vi "test-Diff-Drive-Accel-Limiter-Test1.vi"(8 "error in (no error)":errorcluster) -> (0 "error out":errorcluster, 3 "All tests passed":bool)   [LabVIEW 2019]
uses:
  <vilib>/Rock Robotics/WPI/ThirdParty/JAS_Junk/TrajLib/Trajectory_Library.lvlib
  <vilib>/Analysis/NI_AALBase.lvlib
  <vilib>/Analysis/baseanly.llb/Real A x B.vi
  <vilib>/Analysis/Matrix/NI_Matrix.lvlib
  <vilib>/Analysis/Matrix/Numeric/Add/Add - RM,RM.vi
panel:
  out "max value 6":dbl
  out "max value 5":dbl
  out "max value 4":dbl
  out "max value 3":dbl
  out "max value 2":dbl
  out "max value":dbl
  out "Test 1":bool
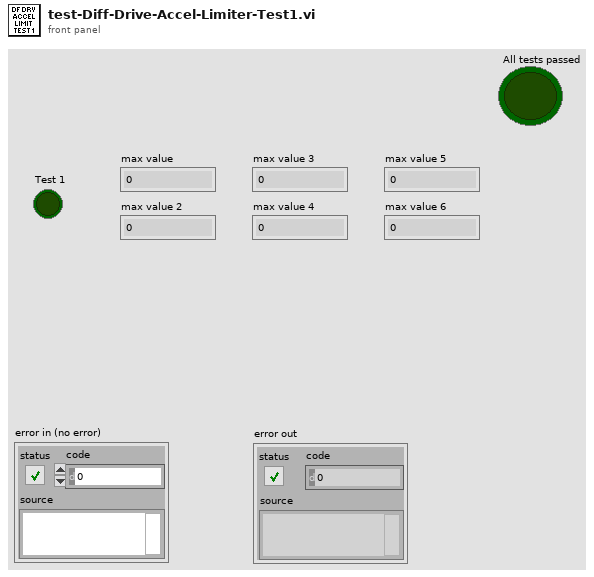
[diagram p1: front panel]
types:
  T1 = typedef "NI_Matrix.lvlib/RealMatrix.ctl" = dbl[][]
  T2 = typedef "Trajectory_Library.lvlib/LINEAR_SYSTEM.ctl" = cluster{"m_A":T1, "m_B":T1, "m_C":T1, "m_D":T1, "States":i32, "Inputs":i32, "Outputs":i32}
  T3 = typedef "Trajectory_Library.lvlib/DIFF_DRIVE_ACCEL_LIMIT.ctl" = cluster{"m_system":T2, "m_trackwidth":dbl, "m_maxLinearAccel":dbl, "m_maxAngularAccel":dbl, "m_minLinearAccel":dbl}
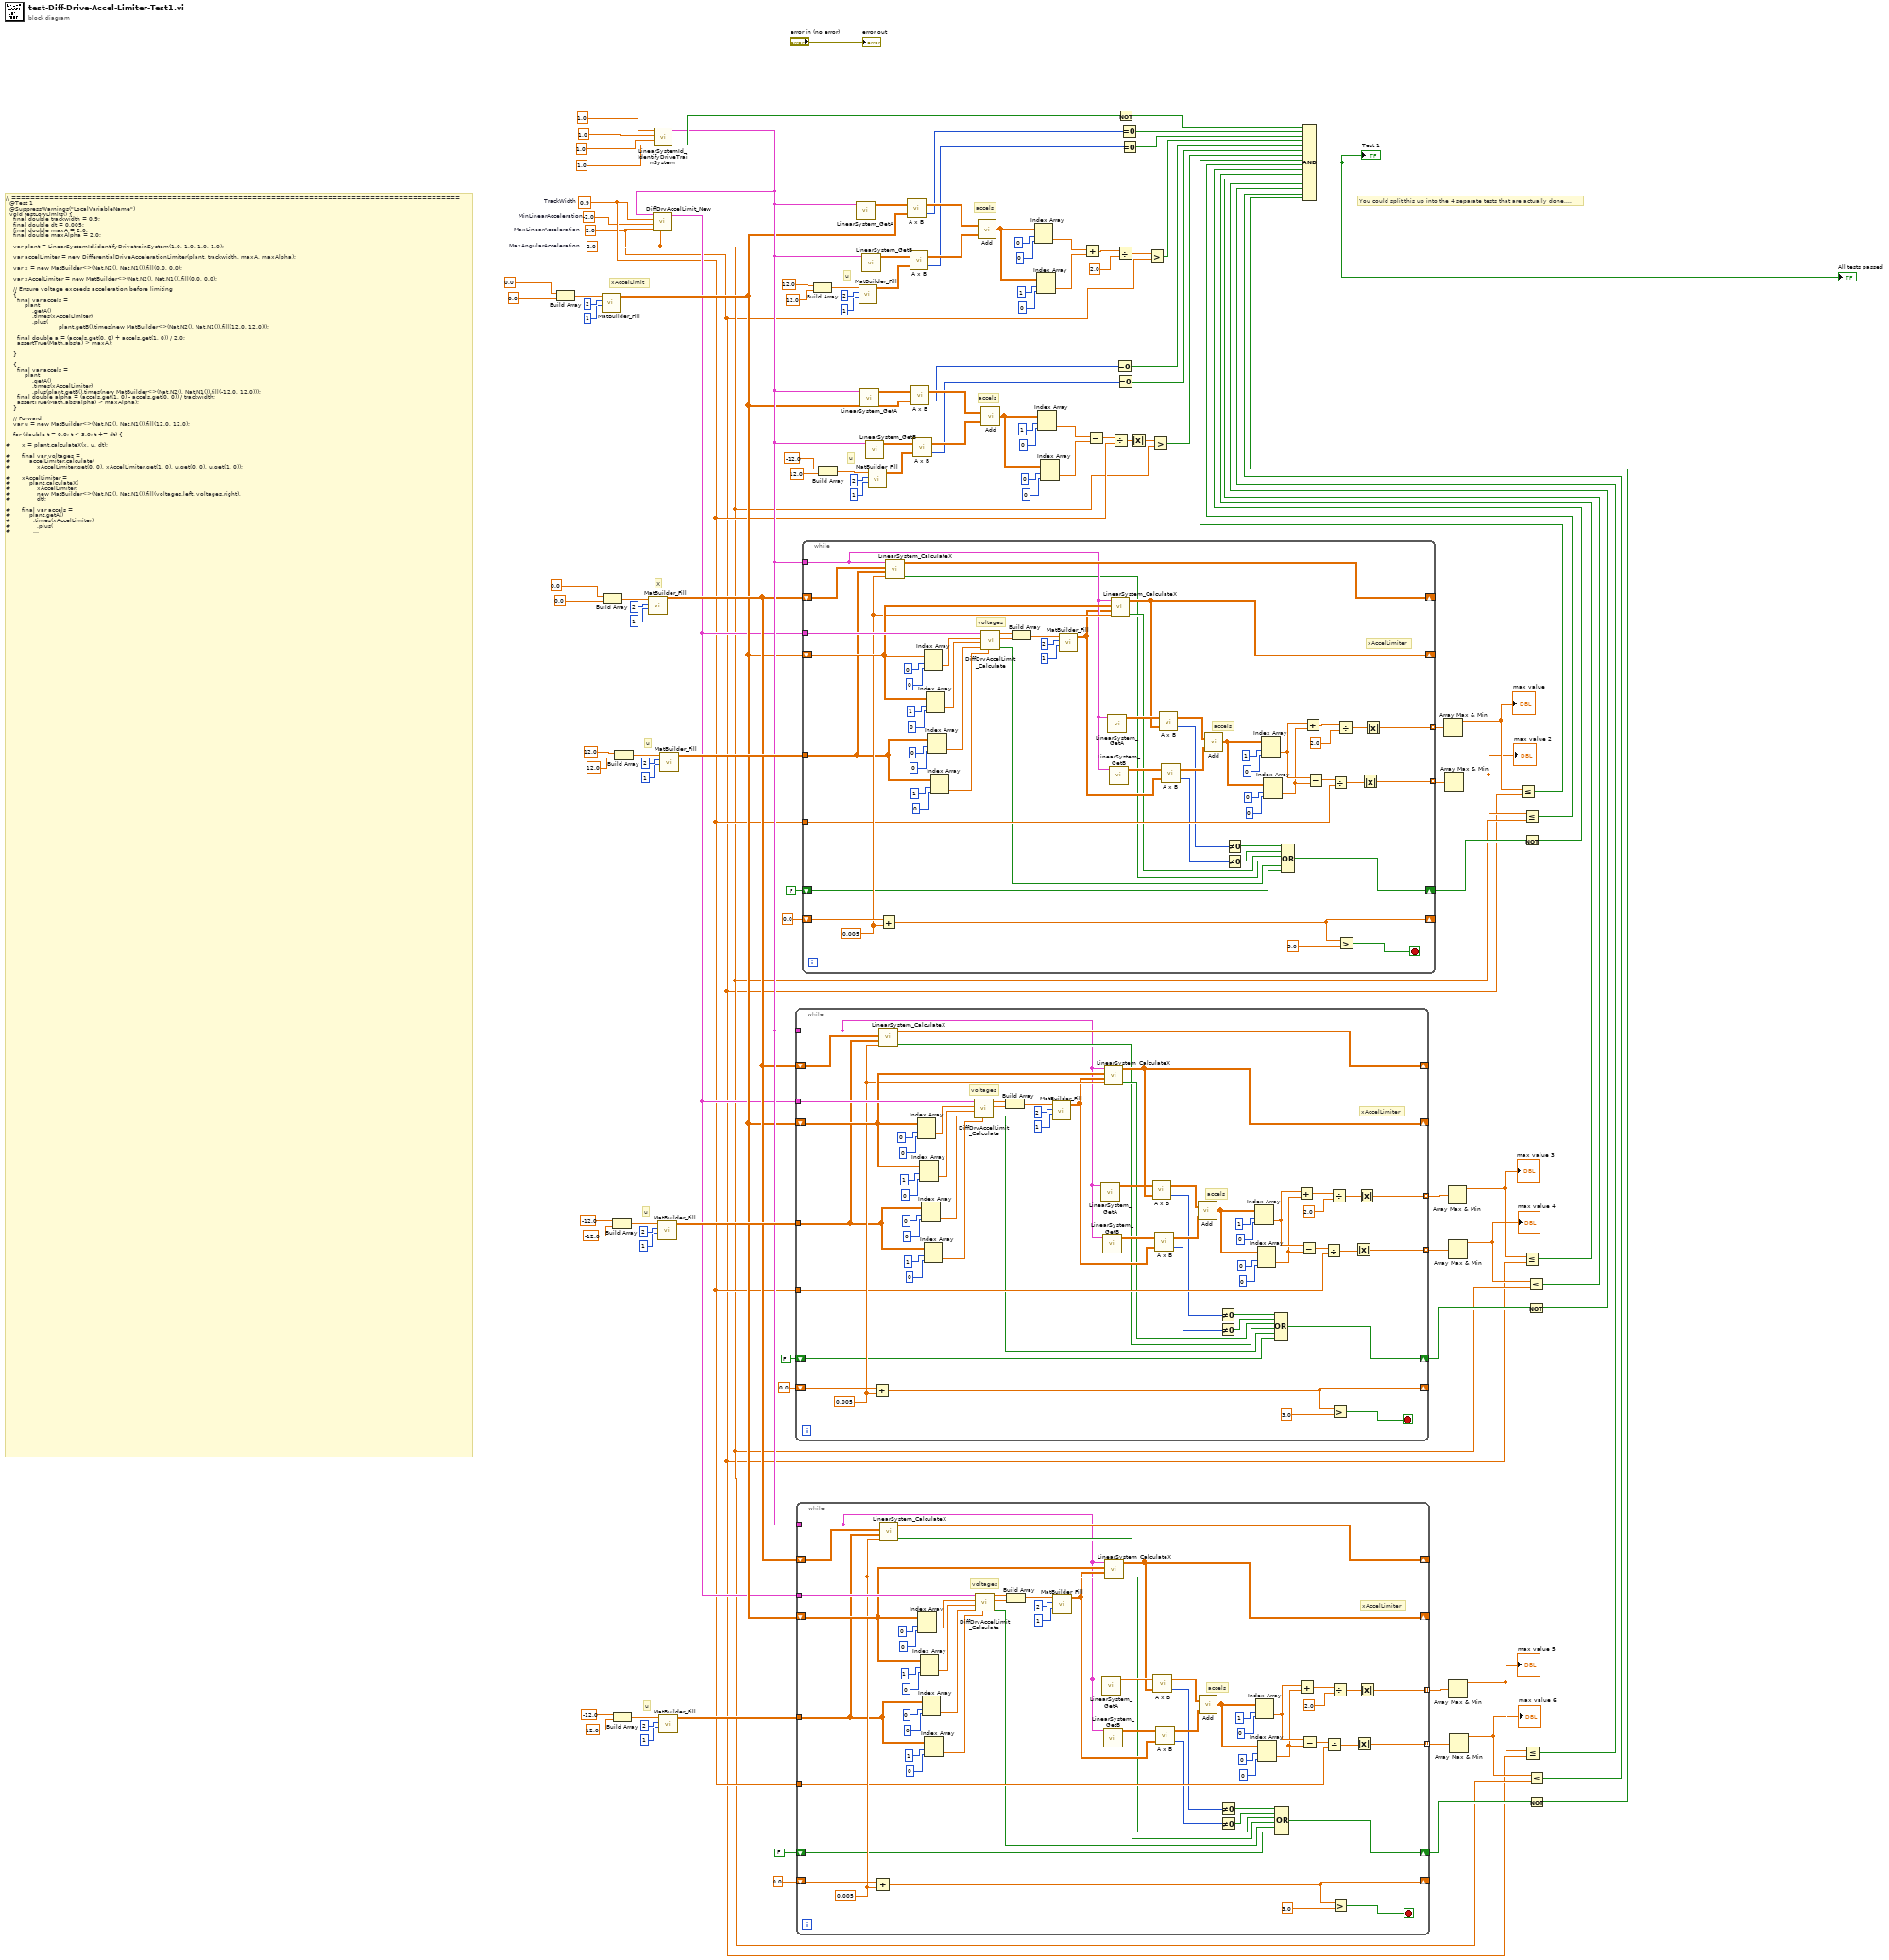
[diagram p0: block diagram]
diagram:
  w1 = -2.0  # MinLinearAcceleration
  w8 = 0.9  # TrackWidth
  w2 = 2.0  # MaxLinearAcceleration
  w3 = 2.0  # MaxAngularAcceleration
  # "You could split this up into the 4 separate tests that are actually done...."
  # "u"
  # "u"
  # "u"
  # "u"
  # "u"
  # "accels"
  # "accels"
  # "xAccelLimit"
  # "X"
  # "// ===============================================================================================\n  @Test 1\n  @SuppressWarnings(\"LocalVariableName\")\n  void testLowLimits() {\n    final double trackwidth = 0.9;\n    final double dt = 0.005;\n    final double maxA = 2.0;\n    final double maxAlpha = 2.0;\n\n    var plant = LinearSystemId.identifyDrivetrainSystem(1.0, 1.0, 1.0, 1.0);\n\n    var accelLimiter = new DifferentialDriveAccelerationLimiter(plant, trackwidth, maxA, maxAlpha);\n\n    var x = new MatBuilder<>(Nat.N2(), Nat.N1()).fill(0.0, 0.0);\n\n    var xAccelLimiter = new MatBuilder<>(Nat.N2(), Nat.N1()).fill(0.0, 0.0);\n\n    // Ensure voltage exceeds acceleration before limiting\n    {\n      final var accels =\n          plant\n              .getA()\n              .times(xAccelLimiter)\n              .plus(\n                            plant.getB().times(new MatBuilder<>(Nat.N2(), Nat.N1()).fill(12.0, 12.0)));\n\n      final double a = (accels.get(0, 0) + accels.get(1, 0)) / 2.0;\n      assertTrue(Math.abs(a) > maxA);\n\n    }\n\n    {\n      final var accels =\n          plant\n              .getA()\n              .times(xAccelLimiter)\n              .plus(plant.getB().times(new MatBuilder<>(Nat.N2(), Nat.N1()).fill(-12.0, 12.0)));\n      final double alpha = (accels.get(1, 0) - accels.get(0, 0)) / trackwidth;\n      assertTrue(Math.abs(alpha) > maxAlpha);\n    }\n\n    // Forward\n    var u = new MatBuilder<>(Nat.N2(), Nat.N1()).fill(12.0, 12.0);\n\n    for (double t = 0.0; t < 3.0; t += dt) {\n\n#      x = plant.calculateX(x, u, dt);\n\n#      final var voltages =\n#          accelLimiter.calculate(\n#              xAccelLimiter.get(0, 0), xAccelLimiter.get(1, 0), u.get(0, 0), u.get(1, 0));\n\n#      xAccelLimiter =\n#          plant.calculateX(\n#              xAccelLimiter,\n#              new MatBuilder<>(Nat.N2(), Nat.N1()).fill(voltages.left, voltages.right),\n#              dt);\n\n#      final var accels =\n#          plant.getA()\n#            .times(xAccelLimiter)\n#              .plus(\n#                  plant.getB()\n#                      .times(\n#                          new MatBuilder<>(Nat.N2(), Nat.N1())\n#                              .fill(voltages.left, voltages.right)));\n\n#      final double a = (accels.get(0, 0) + accels.get(1, 0)) / 2.0;\n\n#      final double alpha = (accels.get(1, 0) - accels.get(0, 0)) / trackwidth;\n\n#      assertTrue(Math.abs(a) <= maxA);\n#      assertTrue(Math.abs(alpha) <= maxAlpha);\n\n#    }\n\n    // Backward\n    u = new MatBuilder<>(Nat.N2(), Nat.N1()).fill(-12.0, -12.0);\n\n    for (double t = 0.0; t < 3.0; t += dt) {\n      x = plant.calculateX(x, u, dt);\n      final var voltages =\n          accelLimiter.calculate(\n              xAccelLimiter.get(0, 0), xAccelLimiter.get(1, 0), u.get(0, 0), u.get(1, 0));\n      xAccelLimiter =\n          plant.calculateX(\n              xAccelLimiter,\n              new MatBuilder<>(Nat.N2(), Nat.N1()).fill(voltages.left, voltages.right),\n              dt);\n\n      final var accels =\n          plant\n              .getA()\n              .times(xAccelLimiter)\n              .plus(\n                  plant\n                      .getB()\n                      .times(\n                          new MatBuilder<>(Nat.N2(), Nat.N1())\n                              .fill(voltages.left, voltages.right)));\n\n      final double a = (accels.get(0, 0) + accels.get(1, 0)) / 2.0;\n\n      final double alpha = (accels.get(1, 0) - accels.get(0, 0)) / trackwidth;\n\n      assertTrue(Math.abs(a) <= maxA);\n      assertTrue(Math.abs(alpha) <= maxAlpha);\n    }\n\n\n    // Rotate CCW\n    u = new MatBuilder<>(Nat.N2(), Nat.N1()).fill(-12.0, 12.0);\n    for (double t = 0.0; t < 3.0; t += dt) {\n      x = plant.calculateX(x, u, dt);\n      final var voltages =\n          accelLimiter.calculate(\n              xAccelLimiter.get(0, 0), xAccelLimiter.get(1, 0), u.get(0, 0), u.get(1, 0));\n      xAccelLimiter =\n          plant.calculateX(\n              xAccelLimiter,\n              new MatBuilder<>(Nat.N2(), Nat.N1()).fill(voltages.left, voltages.right),\n              dt);\n\n      final var accels =\n          plant\n              .getA()\n              .times(xAccelLimiter)\n              .plus(\n                  plant\n                      .getB()\n                      .times(\n                          new MatBuilder<>(Nat.N2(), Nat.N1())\n                              .fill(voltages.left, voltages.right)));\n      final double a = (accels.get(0, 0) + accels.get(1, 0)) / 2.0;\n      final double alpha = (accels.get(1, 0) - accels.get(0, 0)) / trackwidth;\n      assertTrue(Math.abs(a) <= maxA);\n      assertTrue(Math.abs(alpha) <= maxAlpha);\n    }\n  }"
  n1 = Build Array(0.0 ("element"), 0.0 ("element")) -> (w114:dbl[])
  n2 = call <vilib>:"MatBuilder_Fill.vi"("Columns"=1, "Rows"=2, "Value List"=w114) -> ("output matrix"=w10:T1)  [unwired: 8 in]
  n3 = Build Array(0.0 ("element"), 0.0 ("element")) -> (w119:dbl[])
  n4 = Build Array(-12.0 ("element"), -12.0 ("element")) -> (w39:dbl[])
  n5 = Build Array(-12.0 ("element"), 12.0 ("element")) -> (w23:dbl[])
  n6 = Build Array(12.0 ("element"), 12.0 ("element")) -> (w57:dbl[])
  n7 = call <vilib>:"MatBuilder_Fill.vi"("Columns"=1, "Rows"=2, "Value List"=w119) -> ("output matrix"=w11:T1)  [unwired: 8 in]
  n8 = call <vilib>:"LinearSystemId_IdentifyDriveTrainSystem.vi"("kAAngular"=1.0 ("rbMeters"), "kVAngular"=1.0 ("rMeters"), "kALinear"=1.0 ("MassKg"), "kVLinear"=1.0 ("JKgMetersSquared")) -> ("Size Coerced"=w94:bool, "Linearsystem"=w12:T2)  [unwired: 6 in]
  n9 = call <vilib>:"DiffDrvAccelLimit_New.vi"("MaxAngularAcceleration"=w3, "MaxLinearAcceleration"=w2, "MinLinearAcceleration"=w1, "TrackWidth"=w8, "LINEARSYSTEM"=w12) -> ("outDiffDriveAccelLimit"=w9:T3)  [unwired: 5 in, 1 out]
  n10 = call <vilib>:"MatBuilder_Fill.vi"("Columns"=1, "Rows"=2, "Value List"=w39) -> ("output matrix"=w34:T1)  [unwired: 8 in]
  n11 = call <vilib>:"MatBuilder_Fill.vi"("Columns"=1, "Rows"=2, "Value List"=w23) -> ("output matrix"=w18:T1)  [unwired: 8 in]
  n12 = call <vilib>:"MatBuilder_Fill.vi"("Columns"=1, "Rows"=2, "Value List"=w57) -> ("output matrix"=w51:T1)  [unwired: 8 in]
  n13 = while {
    shift-right: [w179] -> _
    shift-left: 0.0 -> [w182]
    tunnel: w34 -> [w140]
    shift-right: [w172] -> _
    shift-left: w11 -> [w178]
    tunnel: w9 -> [w177]
    shift-right: [w147] -> _
    shift-left: w10 -> [w163]
    tunnel: w8 -> [w139]
    tunnel: [w136] -> w31 mode=indexing
    tunnel: [w135] -> w30 mode=indexing
    shift-right: [w126] -> w29
    shift-left: FALSE -> [w127]
    tunnel: w12 -> [w125]
    stop <- w181 stop-if-true
    w157 = 0.005
    # "voltages"
    # "xAccelLimiter"
    # "accels"
    n14 = Add(x=w182, y=w157) -> (x+y=w179:dbl)
    n15 = call <vilib>:"LinearSystem_CalculateX.vi"("dT_Seconds"=w157, "ClampedU"=w140, "X"=w178, "Linearsystem"=w125) -> ("Error"=w129:bool, "outX"=w172:T1)  [unwired: 6 in]
    n16 = Index Array(array=w163, index (row)=0, index (col)=0) -> (element=w171:dbl)
    n17 = Index Array(array=w163, index (row)=1, index (col)=0) -> (element=w170:dbl)
    n18 = Index Array(array=w140, index (row)=0, index (col)=0) -> (element=w165:dbl)
    n19 = Index Array(array=w140, index (row)=1, index (col)=0) -> (element=w164:dbl)
    n20 = call <vilib>:"DiffDrvAccelLimit_Calculate.vi"("RightVoltage"=w164, "LeftVoltage"=w165, "RightVelocity"=w170, "LeftVelocity"=w171, "inDiffDriveAccelLimit"=w177) -> ("Error"=w128:bool, "NewRightVoltage"=w158:dbl, "NewLeftVoltage"=w159:dbl)  [unwired: 4 in]
    n21 = Build Array(w159, w158) -> (w162:dbl[])
    n22 = call <vilib>:"MatBuilder_Fill.vi"("Columns"=1, "Rows"=2, "Value List"=w162) -> ("output matrix"=w146:T1)  [unwired: 8 in]
    n23 = call <vilib>:"LinearSystem_GetA.vi"("Linearsystem"=w125) -> ("A"=w156:T1)  [unwired: 10 in]
    n24 = call <vilib>:"LinearSystem_GetB.vi"("Linearsystem"=w125) -> ("B"=w155:T1)  [unwired: 10 in]
    n25 = call <vilib>:"LinearSystem_CalculateX.vi"("dT_Seconds"=w157, "ClampedU"=w146, "X"=w163, "Linearsystem"=w125) -> ("Error"=w130:bool, "outX"=w147:T1)  [unwired: 6 in]
    n26 = call-poly <vilib>:"A x B.vi"("B"=w147, "A"=w156) -> ("error"=w133:i32, "A x B"=w154:T1)
    n27 = call-poly <vilib>:"A x B.vi"("B"=w146, "A"=w155) -> ("error"=w132:i32, "A x B"=w153:T1)
    n28 = call-poly <vilib>:"Add.vi"("Real Matrix B"=w153, "Real Matrix A"=w154) -> ("A + B"=w148:T1)
    n29 = Not Equal To 0?(x=w133) -> (x != 0?=w134:bool)
    n30 = Not Equal To 0?(x=w132) -> (x != 0?=w131:bool)
    n31 = Index Array(array=w148, index (row)=1, index (col)=0) -> (element=w142:dbl)
    n32 = Index Array(array=w148, index (row)=0, index (col)=0) -> (element=w141:dbl)
    n33 = Compound Arithmetic op=OR(w134, w131, w130, w129, w128, w127) -> (w126:bool)
    n34 = Add(x=w142, y=w141) -> (x+y=w145:dbl)
    n35 = Subtract(x=w142, y=w141) -> (x-y=w143:dbl)
    n36 = Divide(x=w143, y=w139) -> (x/y=w137:dbl)
    n37 = Divide(x=w145, y=2.0) -> (x/y=w138:dbl)
    n38 = Greater?(x=w179, y=3.0) -> (0:w181:bool)
    n39 = Absolute Value(x=w137) -> (abs(x)=w135:dbl)
    n40 = Absolute Value(x=w138) -> (abs(x)=w136:dbl)
  }
  n41 = while {
    shift-right: [w237] -> _
    shift-left: 0.0 -> [w240]
    tunnel: w18 -> [w198]
    shift-right: [w230] -> _
    shift-left: w11 -> [w236]
    tunnel: w9 -> [w235]
    shift-right: [w205] -> _
    shift-left: w10 -> [w221]
    tunnel: w8 -> [w197]
    tunnel: [w194] -> w15 mode=indexing
    tunnel: [w193] -> w14 mode=indexing
    shift-right: [w184] -> w13
    shift-left: FALSE -> [w185]
    tunnel: w12 -> [w183]
    stop <- w239 stop-if-true
    w215 = 0.005
    # "voltages"
    # "xAccelLimiter"
    # "accels"
    n42 = Add(x=w240, y=w215) -> (x+y=w237:dbl)
    n43 = call <vilib>:"LinearSystem_CalculateX.vi"("dT_Seconds"=w215, "ClampedU"=w198, "X"=w236, "Linearsystem"=w183) -> ("Error"=w187:bool, "outX"=w230:T1)  [unwired: 6 in]
    n44 = Index Array(array=w221, index (row)=0, index (col)=0) -> (element=w229:dbl)
    n45 = Index Array(array=w221, index (row)=1, index (col)=0) -> (element=w228:dbl)
    n46 = Index Array(array=w198, index (row)=0, index (col)=0) -> (element=w223:dbl)
    n47 = Index Array(array=w198, index (row)=1, index (col)=0) -> (element=w222:dbl)
    n48 = call <vilib>:"DiffDrvAccelLimit_Calculate.vi"("RightVoltage"=w222, "LeftVoltage"=w223, "RightVelocity"=w228, "LeftVelocity"=w229, "inDiffDriveAccelLimit"=w235) -> ("Error"=w186:bool, "NewRightVoltage"=w216:dbl, "NewLeftVoltage"=w217:dbl)  [unwired: 4 in]
    n49 = Build Array(w217, w216) -> (w220:dbl[])
    n50 = call <vilib>:"MatBuilder_Fill.vi"("Columns"=1, "Rows"=2, "Value List"=w220) -> ("output matrix"=w204:T1)  [unwired: 8 in]
    n51 = call <vilib>:"LinearSystem_GetA.vi"("Linearsystem"=w183) -> ("A"=w214:T1)  [unwired: 10 in]
    n52 = call <vilib>:"LinearSystem_GetB.vi"("Linearsystem"=w183) -> ("B"=w213:T1)  [unwired: 10 in]
    n53 = call <vilib>:"LinearSystem_CalculateX.vi"("dT_Seconds"=w215, "ClampedU"=w204, "X"=w221, "Linearsystem"=w183) -> ("Error"=w188:bool, "outX"=w205:T1)  [unwired: 6 in]
    n54 = call-poly <vilib>:"A x B.vi"("B"=w205, "A"=w214) -> ("error"=w191:i32, "A x B"=w212:T1)
    n55 = call-poly <vilib>:"A x B.vi"("B"=w204, "A"=w213) -> ("error"=w190:i32, "A x B"=w211:T1)
    n56 = call-poly <vilib>:"Add.vi"("Real Matrix B"=w211, "Real Matrix A"=w212) -> ("A + B"=w206:T1)
    n57 = Not Equal To 0?(x=w191) -> (x != 0?=w192:bool)
    n58 = Not Equal To 0?(x=w190) -> (x != 0?=w189:bool)
    n59 = Index Array(array=w206, index (row)=1, index (col)=0) -> (element=w200:dbl)
    n60 = Index Array(array=w206, index (row)=0, index (col)=0) -> (element=w199:dbl)
    n61 = Compound Arithmetic op=OR(w192, w189, w188, w187, w186, w185) -> (w184:bool)
    n62 = Add(x=w200, y=w199) -> (x+y=w203:dbl)
    n63 = Subtract(x=w200, y=w199) -> (x-y=w201:dbl)
    n64 = Divide(x=w201, y=w197) -> (x/y=w195:dbl)
    n65 = Divide(x=w203, y=2.0) -> (x/y=w196:dbl)
    n66 = Greater?(x=w237, y=3.0) -> (0:w239:bool)
    n67 = Absolute Value(x=w195) -> (abs(x)=w193:dbl)
    n68 = Absolute Value(x=w196) -> (abs(x)=w194:dbl)
  }
  n69 = while {
    shift-right: [w295] -> _
    shift-left: 0.0 -> [w298]
    tunnel: w12 -> [w263]
    tunnel: w51 -> [w255]
    shift-right: [w288] -> _
    shift-left: w11 -> [w294]
    tunnel: w9 -> [w293]
    shift-right: [w262] -> _
    shift-left: w10 -> [w279]
    tunnel: w8 -> [w254]
    tunnel: [w251] -> w50 mode=indexing
    tunnel: [w250] -> w49 mode=indexing
    shift-right: [w241] -> w45
    shift-left: FALSE -> [w242]
    stop <- w297 stop-if-true
    w273 = 0.005
    # "voltages"
    # "xAccelLimiter"
    # "accels"
    n70 = Add(x=w298, y=w273) -> (x+y=w295:dbl)
    n71 = call <vilib>:"LinearSystem_CalculateX.vi"("dT_Seconds"=w273, "ClampedU"=w255, "X"=w294, "Linearsystem"=w263) -> ("Error"=w244:bool, "outX"=w288:T1)  [unwired: 6 in]
    n72 = Index Array(array=w279, index (row)=0, index (col)=0) -> (element=w287:dbl)
    n73 = Index Array(array=w279, index (row)=1, index (col)=0) -> (element=w286:dbl)
    n74 = Index Array(array=w255, index (row)=0, index (col)=0) -> (element=w281:dbl)
    n75 = Index Array(array=w255, index (row)=1, index (col)=0) -> (element=w280:dbl)
    n76 = call <vilib>:"DiffDrvAccelLimit_Calculate.vi"("RightVoltage"=w280, "LeftVoltage"=w281, "RightVelocity"=w286, "LeftVelocity"=w287, "inDiffDriveAccelLimit"=w293) -> ("Error"=w243:bool, "NewRightVoltage"=w274:dbl, "NewLeftVoltage"=w275:dbl)  [unwired: 4 in]
    n77 = Build Array(w275, w274) -> (w278:dbl[])
    n78 = call <vilib>:"MatBuilder_Fill.vi"("Columns"=1, "Rows"=2, "Value List"=w278) -> ("output matrix"=w261:T1)  [unwired: 8 in]
    n79 = call <vilib>:"LinearSystem_GetA.vi"("Linearsystem"=w263) -> ("A"=w272:T1)  [unwired: 10 in]
    n80 = call <vilib>:"LinearSystem_GetB.vi"("Linearsystem"=w263) -> ("B"=w271:T1)  [unwired: 10 in]
    n81 = call <vilib>:"LinearSystem_CalculateX.vi"("dT_Seconds"=w273, "ClampedU"=w261, "X"=w279, "Linearsystem"=w263) -> ("Error"=w245:bool, "outX"=w262:T1)  [unwired: 6 in]
    n82 = call-poly <vilib>:"A x B.vi"("B"=w262, "A"=w272) -> ("error"=w248:i32, "A x B"=w270:T1)
    n83 = call-poly <vilib>:"A x B.vi"("B"=w261, "A"=w271) -> ("error"=w247:i32, "A x B"=w269:T1)
    n84 = call-poly <vilib>:"Add.vi"("Real Matrix B"=w269, "Real Matrix A"=w270) -> ("A + B"=w264:T1)
    n85 = Not Equal To 0?(x=w248) -> (x != 0?=w249:bool)
    n86 = Not Equal To 0?(x=w247) -> (x != 0?=w246:bool)
    n87 = Index Array(array=w264, index (row)=1, index (col)=0) -> (element=w257:dbl)
    n88 = Index Array(array=w264, index (row)=0, index (col)=0) -> (element=w256:dbl)
    n89 = Compound Arithmetic op=OR(w249, w246, w245, w244, w243, w242) -> (w241:bool)
    n90 = Add(x=w257, y=w256) -> (x+y=w260:dbl)
    n91 = Subtract(x=w257, y=w256) -> (x-y=w258:dbl)
    n92 = Divide(x=w258, y=w254) -> (x/y=w252:dbl)
    n93 = Divide(x=w260, y=2.0) -> (x/y=w253:dbl)
    n94 = Greater?(x=w295, y=3.0) -> (0:w297:bool)
    n95 = Absolute Value(x=w252) -> (abs(x)=w250:dbl)
    n96 = Absolute Value(x=w253) -> (abs(x)=w251:dbl)
  }
  n97 = Build Array(12.0 ("element"), 12.0 ("element")) -> (w107:dbl[])
  n98 = Build Array(-12.0 ("element"), 12.0 ("element")) -> (w70:dbl[])
  n99 = call <vilib>:"LinearSystem_GetA.vi"("Linearsystem"=w12) -> ("A"=w109:T1)  [unwired: 10 in]
  n100 = call <vilib>:"MatBuilder_Fill.vi"("Columns"=1, "Rows"=2, "Value List"=w107) -> ("output matrix"=w102:T1)  [unwired: 8 in]
  n101 = call <vilib>:"LinearSystem_GetA.vi"("Linearsystem"=w12) -> ("A"=w82:T1)  [unwired: 10 in]
  n102 = call <vilib>:"LinearSystem_GetB.vi"("Linearsystem"=w12) -> ("B"=w108:T1)  [unwired: 10 in]
  n103 = call <vilib>:"LinearSystem_GetB.vi"("Linearsystem"=w12) -> ("B"=w81:T1)  [unwired: 10 in]
  n104 = call <vilib>:"MatBuilder_Fill.vi"("Columns"=1, "Rows"=2, "Value List"=w70) -> ("output matrix"=w65:T1)  [unwired: 8 in]
  n105 = call-poly <vilib>:"A x B.vi"("B"=w10, "A"=w109) -> ("error"=w92:i32, "A x B"=w101:T1)
  n106 = call-poly <vilib>:"A x B.vi"("B"=w102, "A"=w108) -> ("error"=w91:i32, "A x B"=w100:T1)
  n107 = call-poly <vilib>:"A x B.vi"("B"=w10, "A"=w82) -> ("error"=w64:i32, "A x B"=w80:T1)
  n108 = call-poly <vilib>:"A x B.vi"("B"=w65, "A"=w81) -> ("error"=w63:i32, "A x B"=w79:T1)
  n109 = call-poly <vilib>:"Add.vi"("Real Matrix B"=w100, "Real Matrix A"=w101) -> ("A + B"=w95:T1)
  n110 = call-poly <vilib>:"Add.vi"("Real Matrix B"=w79, "Real Matrix A"=w80) -> ("A + B"=w74:T1)
  n111 = Index Array(array=w95, index (row)=0, index (col)=0) -> (element=w88:dbl)
  n112 = Index Array(array=w95, index (row)=1, index (col)=0) -> (element=w87:dbl)
  n113 = Index Array(array=w74, index (row)=1, index (col)=0) -> (element=w73:dbl)
  n114 = Index Array(array=w74, index (row)=0, index (col)=0) -> (element=w72:dbl)
  n115 = Add(x=w88, y=w87) -> (x+y=w86:dbl)
  n116 = Subtract(x=w73, y=w72) -> (x-y=w71:dbl)
  n117 = Divide(x=w71, y=w8) -> (x/y=w62:dbl)
  n118 = Equal To 0?(x=w64) -> (x = 0?=w60:bool)
  n119 = Divide(x=w86, y=2.0) -> (x/y=w84:dbl)
  n120 = Equal To 0?(x=w63) -> (x = 0?=w59:bool)
  n121 = Not(x=w94) -> (.not. x?=w93:bool)
  n122 = Equal To 0?(x=w92) -> (x = 0?=w90:bool)
  n123 = Equal To 0?(x=w91) -> (x = 0?=w89:bool)
  n124 = Absolute Value(x=w62) -> (abs(x)=w61:dbl)
  n125 = Greater?(x=w84, y=w2) -> (0:w83:bool)
  n126 = Greater?(x=w61, y=w3) -> (0:w58:bool)
  n127 = Array Max & Min(array=w50) -> (max value=w48:dbl)  [unwired: 3 out]
  "max value" <- w48
  n128 = Array Max & Min(array=w49) -> (max value=w47:dbl)  [unwired: 3 out]
  "max value 2" <- w47
  n129 = Array Max & Min(array=w31) -> (max value=w33:dbl)  [unwired: 3 out]
  "max value 3" <- w33
  n130 = Array Max & Min(array=w30) -> (max value=w32:dbl)  [unwired: 3 out]
  "max value 4" <- w32
  n131 = Array Max & Min(array=w15) -> (max value=w17:dbl)  [unwired: 3 out]
  "max value 5" <- w17
  n132 = Array Max & Min(array=w14) -> (max value=w16:dbl)  [unwired: 3 out]
  "max value 6" <- w16
  n133 = Less Or Equal?(x=w48, y=w2) -> (x <= y?=w44:bool)
  n134 = Less Or Equal?(x=w47, y=w3) -> (x <= y?=w43:bool)
  n135 = Not(x=w45) -> (.not. x?=w42:bool)
  n136 = Less Or Equal?(x=w33, y=w2) -> (x <= y?=w28:bool)
  n137 = Less Or Equal?(x=w17, y=w2) -> (x <= y?=w7:bool)
  n138 = Less Or Equal?(x=w32, y=w3) -> (x <= y?=w27:bool)
  n139 = Not(x=w29) -> (.not. x?=w26:bool)
  n140 = Less Or Equal?(x=w16, y=w3) -> (x <= y?=w6:bool)
  n141 = Not(x=w13) -> (.not. x?=w5:bool)
  n142 = Compound Arithmetic op=AND(w93, w90, w89, w83, w60, w59, w58, w44, w43, w42, w28, w27, w26, w7, w6, w5) -> (→"All tests passed" →"Test 1":bool)
  "error out" <- "error in (no error)"
